vi "omni_equations.vi"(11 "v=(v_r,v_t,Rw)'":T1) -> (2 "m=D*v=(v1,v2,v3,v4)":T1, 3 "Matrix D":T1=[[-52.0, 0.0, 1.0], [-52.0, 0.0, 1.0], [0.0, 0.0, 1.0], [0.0, 0.0, 1.0]])   [LabVIEW 2016]
uses:
  <vilib>/Analysis/Matrix/Datatypes/RealMatrix.ctl
  <vilib>/Analysis/Matrix/Numeric/Multiply/Multiply - RM,RM.vi
  <vilib>/Analysis/Matrix/Numeric/Conversions/Array To Matrix - RA.vi
  <vilib>/Analysis/Matrix/NI_Matrix.lvlib
panel:
  out "velocidade\ndo robo\ncorrigida":T1
  in  "Matriz m\nobservada":T1
  out "m sem \ndeslizamento \ne no \nsentido \noriginal":dbl[](array[numeric])
  out "deslizamento?":bool
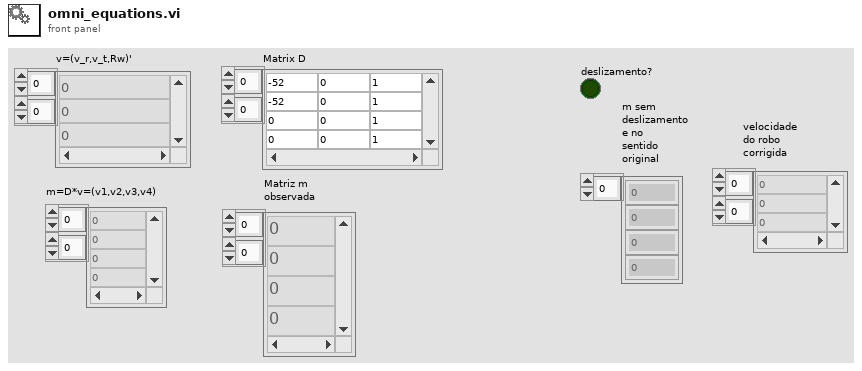
[diagram p1: front panel]
types:
  T1 = typedef "NI_Matrix.lvlib/RealMatrix.ctl" = dbl[][]
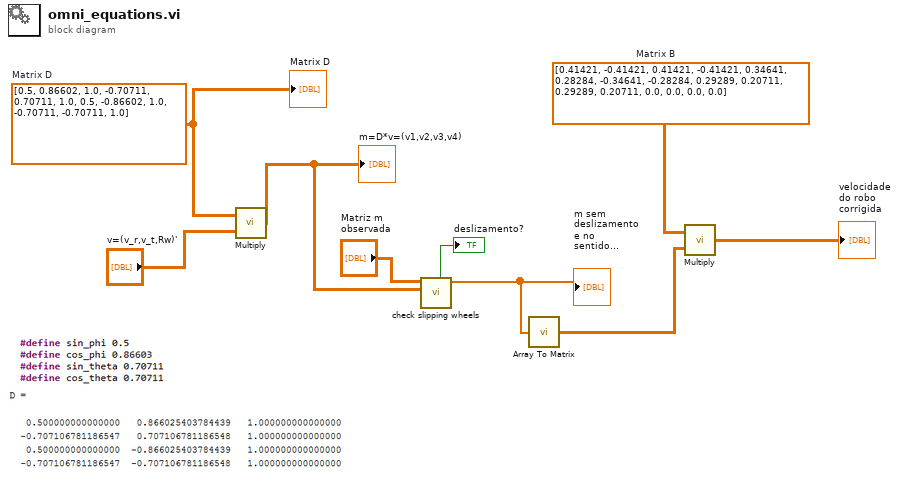
[diagram p0: block diagram]
diagram:
  w4 = T1 [[0.41421, -0.41421, 0.41421, -0.41421], [0.34641, 0.28284, -0.34641, -0.28284], [0.29289, 0.20711, 0.29289, 0.20711], [0.0, 0.0, 0.0, 0.0]]  # Matrix B
  w9 = T1 [[0.5, 0.86602, 1.0], [-0.70711, 0.70711, 1.0], [0.5, -0.86602, 1.0], [-0.70711, -0.70711, 1.0]]  # Matrix D
  n1 = call-poly <vilib>:"Multiply.vi"("Real Matrix B"="v=(v_r,v_t,Rw)'", "Real Matrix A"=w9) -> ("A * B"=w7:T1)
  "m=D*v=(v1,v2,v3,v4)" <- w7
  n2 = call "check slipping wheels.vi"("Matriz m \nesperada"=w7, "Matriz m\nobservada"="Matriz m\nobservada") -> ("m sem \ndeslizamento \ne no \nsentido \noriginal"=w1:dbl[], "deslizamento?"=→"deslizamento?":bool)  [unwired: 7 in, 1 out]
  "m sem \ndeslizamento \ne no \nsentido \noriginal" <- w1
  n3 = call-poly <vilib>:"Array To Matrix.vi"("Real 1D Array"=w1) -> ("Real Matrix (Column Vector)"=w5:T1)
  n4 = call-poly <vilib>:"Multiply.vi"("Real Matrix B"=w5, "Real Matrix A"=w4) -> ("A * B"=→"velocidade\ndo robo\ncorrigida":T1)
  "Matrix D" <- w9
